vi "Change_tip_signal.vi"(8 "error in (no error)":errorcluster, 10 "l_Litho_modes":i32(ring) caption="Ring" items=["Current Measurement ", "Voltage Source", "Direct from BNC"], 11 "Application":refnum<k7>) -> (0 "error out":errorcluster)   [LabVIEW 2016]
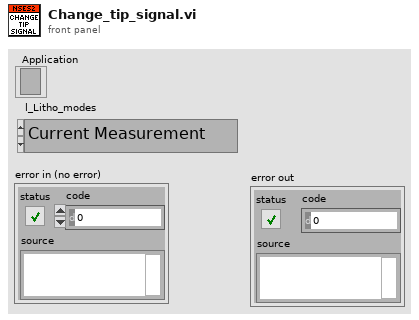
[diagram p1: front panel]
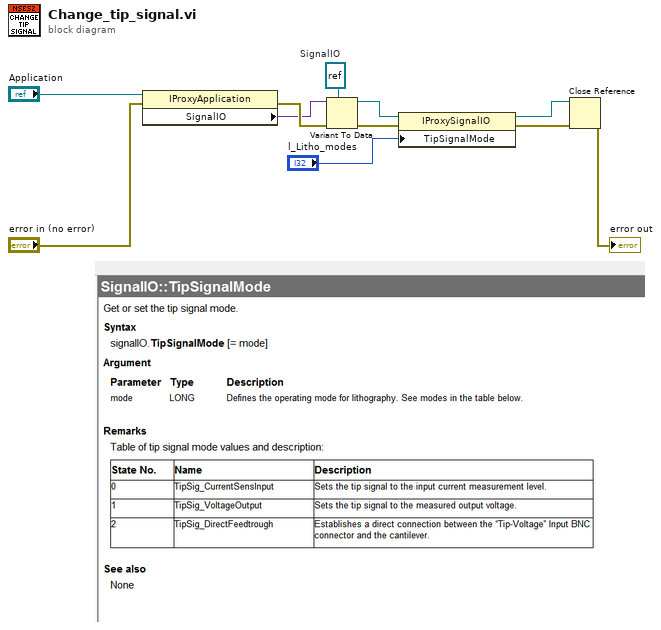
[diagram p0: block diagram]
diagram:
  w9 = refnum<k7> refnum  # SignalIO
  n1 = property class="IProxyApplication"(reference="Application", error in="error in (no error)") -> (error out=w6:errorcluster, "SignalIO"=w3:variant)  [unwired: 1 out]
  n2 = Variant To Data(error in=w6, type=w9, Variant=w3) -> (data=w10:refnum<k7>, error out=w5:errorcluster)
  n3 = property class="IProxySignalIO"(reference=w10, error in=w5, "TipSignalMode"="l_Litho_modes") -> (reference out=w7:refnum<k7>, error out=w4:errorcluster)
  n4 = Close Reference(reference=w7, error in (no error)=w4) -> (error out=→"error out":errorcluster)
